vi "send load from file.vi"(8 "error in":errorcluster, 9 "target alias":string, 10 "tokenized path":T1, 11 "message queue in":T2) -> (0 "error out":errorcluster, 3 "message queue out":T2)   [LabVIEW 2013, in "DCAF Execution Service.lvlib"]
uses:
  DCAF Execution Service.lvlib
  <vilib>/NI/AMC/Message Queue.ctl
  <vilib>/NI/AMC/Message.ctl
  <vilib>/NI/Tools/Keyed Array/KeyedArray.ctl
  tokenized path.ctl
  command commands to rtexe process.ctl
  <vilib>/NI/AMC/Create Single Message.vi
  <vilib>/NI/AMC/Update Message Routing Info.vi
  <vilib>/NI/AMC/Send Message.vi
  <vilib>/NI/AMC/AMC.lvlib
  <vilib>/NI/Tools/Keyed Array/Tools_KeyedArray.lvlib
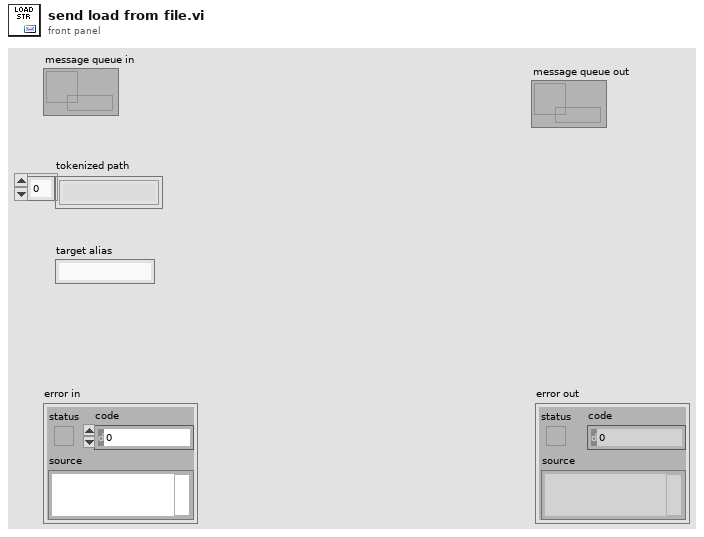
[diagram p1: front panel]
types:
  T1 = typedef "DCAF Execution Service.lvlib/tokenized path.ctl" = string[]
  T2 = typedef "AMC.lvlib/Message Queue.ctl" = refnum<queue>
  T3 = typedef "DCAF Execution Service.lvlib/command commands to rtexe process.ctl" = enum16{"Initialize", "Add Search Paths", "Load from File", "Unload File", "Open All Engines", "Open Single Engine", "Initialize All Engines", "Initialize Single Engine", "Start All", "Start Single", "Pause All", "Pause Single", "Stop All", "Stop Single", "Close All", "Close Single", "Set Safe State All", "Set Safe State Single", "Get Status", "Exit", "Error", "Load Bitfile", "Unload Bitfile", "Clear Faults Single", "Clear Faults All"}
  T4 = cluster{"tokenized path":T1, "target alias":string}
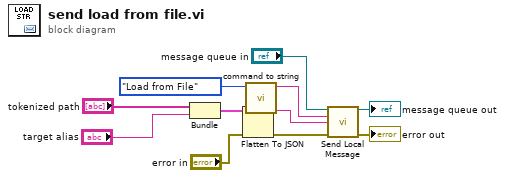
[diagram p0: block diagram]
diagram:
  n1 = Bundle("tokenized path"="tokenized path", "target alias"="target alias") -> (w3:T4)  [unwired: 1 in]
  n2 = Flatten To JSON(anything=w3, error in (no error)="error in") -> (JSON string=w4:string, 11:w5:errorcluster)  [unwired: 1 in]
  n3 = call "command to string.vi"("commands"=command_commands_to_rtexe_process."Load from File") -> ("command string"=w7:string)  [unwired: 10 in]
  n4 = call <vilib>:"Send Local Message.vi"("message queue in"="message queue in", "message name"=w7, "message value"=w4, "error in"=w5) -> ("message queue out"=→"message queue out":T2, "error out"=→"error out":errorcluster)  [unwired: 9 in, 1 out]
